vi "Check Host Software Installed.vi"(8 "error in":errorcluster) -> (0 "error out":errorcluster)   [LabVIEW 2019, in "SEECD System Explorer.lvlib"]
uses:
  SEECD System Explorer.lvlib
  <vilib>/registry/registry.llb/Registry SAM.ctl
  <vilib>/registry/registry.llb/Registry RtKey.ctl
  <vilib>/registry/registry.llb/Read Registry Value Simple STR.vi
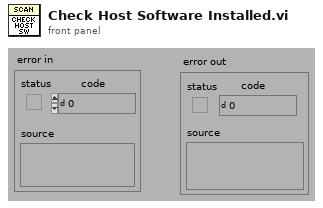
[diagram p1: front panel]
types:
  T1 = typedef "Registry SAM.ctl" = enum32{"KEY_QUERY_VALUE", "KEY_SET_VALUE", "KEY_CREATE_SUB_KEY", "KEY_ENUMERATE_SUB_KEYS", "KEY_NOTIFY", "KEY_CREATE_LINK", "KEY_READ", "KEY_WRITE", "KEY_ALL_ACCESS", "KEY_READ | KEY_WRITE"}
  T2 = typedef "Registry RtKey.ctl" = enum32{"HKEY_CLASSES_ROOT", "HKEY_CURRENT_USER", "HKEY_LOCAL_MACHINE", "HKEY_USERS", "HKEY_PERFORMANCE_DATA", "HKEY_CURRENT_CONFIG", "HKEY_DYN_DATA"}
  T3 = typedef "Registry refnum.ctl" = refnum<k1>
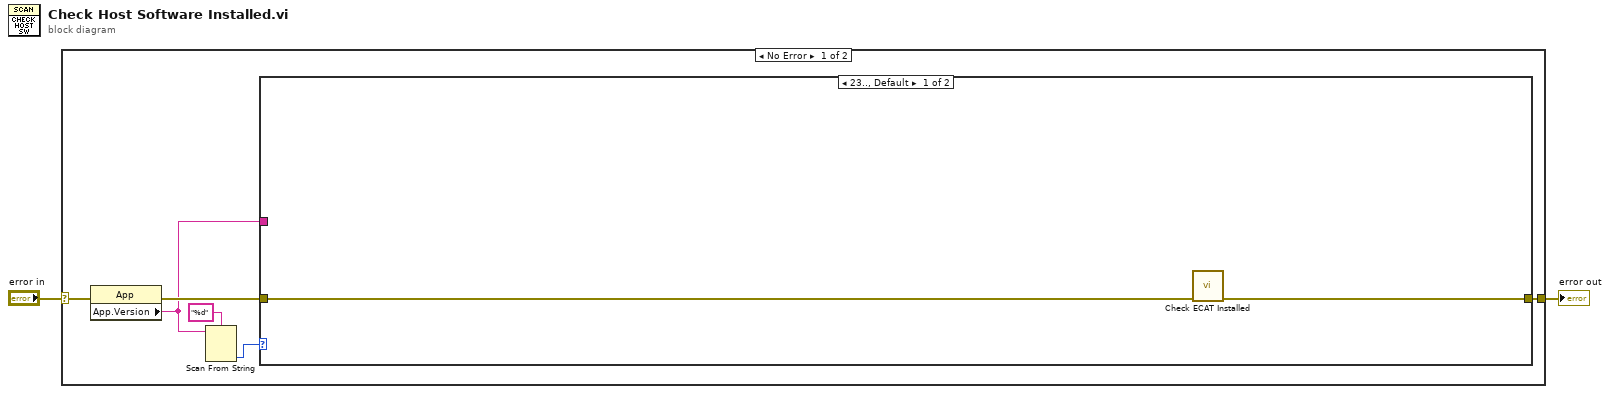
[diagram p0: block diagram]
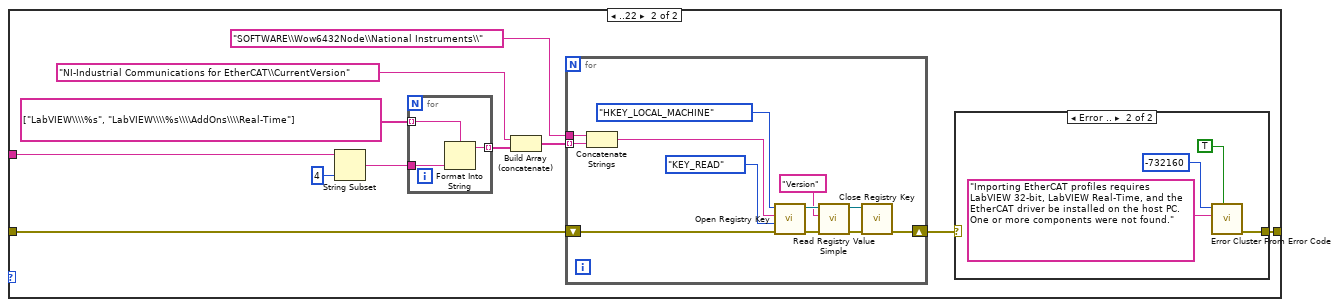
[diagram p2: hidden frame]
diagram:
  n1 = case shown="No Error" "error in" {
    selector: "error in" -> [w6 w42]
    tunnel: [w8 w42] -> w2
    frame No Error {
      n2 = property class="App"(error in=w6) -> (error out=w5:errorcluster, "App.Version"=w3:string)  [unwired: 1 in, 1 out]
      n3 = Scan From String(format string="%d", input string=w3) -> (output 1=w4:i32)  [unwired: 3 in, 3 out]
      n4 = case shown="23.., Default" w4 {
        tunnel: [w10 w13] -> w8
        tunnel: w5 -> [w9 w12]
        tunnel: w3 -> [_ w11]
        frame 23.., Default {
          n5 = call "Check ECAT Installed.vi"("error in (no error)"=w9) -> ("error out"=w10:errorcluster)  [unwired: 10 in]
        }
        frame ..22 {
          n6 = String Subset(string=w11, length (rest)=4 ("length (rest)")) -> (substring=w18:string)  [unwired: 1 in]
          n7 = for {
            tunnel: w18 -> [w29]
            tunnel: string[] ["LabVIEW\\\\%s", "LabVIEW\\\\%s\\\\AddOns\\\\Real-Time"] -> [w27] mode=indexing
            tunnel: [w28] -> w16 mode=indexing
            n8 = Format Into String(format string=w27, w29) -> (resulting string=w28:string)  [unwired: 2 in, 1 out]
          }
          n9 = Build Array (concatenate)("NI-Industrial Communications for EtherCAT\\CurrentVersion", w16) -> (w20:string[])
          n10 = for {
            tunnel: w20 -> [w32] mode=indexing
            shift-right: [w35] -> w14
            shift-left: w12 -> [w33]
            tunnel: "SOFTWARE\\Wow6432Node\\National Instruments\\" -> [w30]
            n11 = Concatenate Strings(w30, w32) -> (w31:string)
            n12 = call <vilib>:"Open Registry Key.vi"("error in (no error)"=w33, "security access mask (KEY_READ | KEY_WRITE)"=Registry_SAM."KEY_READ", "subkey"=w31, "root key (HKEY_LOCAL_MACHINE)"=Registry_RtKey."HKEY_LOCAL_MACHINE") -> ("error out"=w37:errorcluster, "refnum out"=w36:T3)  [unwired: 6 in]
            n13 = call-poly <vilib>:"Read Registry Value Simple.vi"("error in (no error)"=w37, "value"="Version", "refnum"=w36) -> ("error out"=w41:errorcluster, "refnum out"=w40:T3)  [unwired: 3 in, 2 out]
            n14 = call <vilib>:"Close Registry Key.vi"("error in (no error)"=w41, "refnum"=w40) -> ("error out"=w35:errorcluster)  [unwired: 5 in]
          }
          n15 = case shown="Error .." w14 {
            selector: w14 -> [w22 _]
            tunnel: [w22 w23] -> w13
            frame No Error {
            }
            frame Error {
              n16 = call <vilib>:"Error Cluster From Error Code.vi"("show call chain? (False)"=TRUE, "error message (\"\")"="Importing EtherCAT profiles requires LabVIEW 32-bit, LabVIEW Real-Time, and the EtherCAT driver be installed on the host PC. One or more components were not found." ("error message (\"\")"), "error code (0)"=-732160) -> ("error out"=w23:errorcluster)  [unwired: 6 in]
            }
          }
        }
      }
    }
    frame Error {
    }
  }
  "error out" <- w2
